vi "Benchmark SV Receive LV2012 - NI Verified - 100 Byte - 1Var.vi"() -> ()   [LabVIEW 2015]
uses:
  <vilib>/Platform/TimedLoop/XDataNode/timing_clust.ctl
  <vilib>/Platform/TimedLoop/XDataNode/nitl_modes.ctl
  <vilib>/Platform/TimedLoop/XDataNode/wakeup.ctl
  <vilib>/platform/TimedLoop/XDataNode/XDataNode.xnode
  <vilib>/Platform/TimedLoop/XDataNode/XDNodeRunTimeDep.lvlib
panel:
  out "Time":u32
  out "Counter":i32
  out "100 byte":i32[][](array[numeric])
  # "Overview:  Coding that exemplifies how to benchmark the communication of Shared Variables.\nRequirements: LabVIEW 2012 or compatible\nInstructions:\n1. Run this VI\n2. Watch the amount of time it takes to communicate on the \"Benchmark SV Send  LV2012 - NI Verified.vi\" \n3. Stop both VIs"
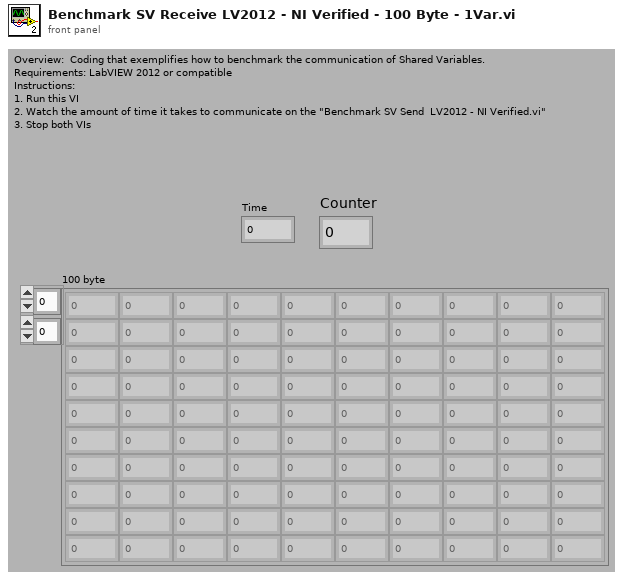
[diagram p1: front panel]
types:
  T1 = typedef "XDNodeRunTimeDep.lvlib/timing_clust.ctl" = cluster{"Expected End [f-1]":u64, "Actual End [f-1]":u64, "Finished Late? [f-1]":bool, "Expected End [i-1]":u64, "Actual End [i-1]":u64, "Finished Late? [i-1]":bool, "Expected Start [i]":u64, "Actual Start [i]":u64, "Expected Start [f]":u64, "Actual Start [f]":u64, "Source Name":string, "Structure Name":string, "Period":i64, "Deadline":i64, "Offset":i64, "Start":i64, "Priority":i32, "Timeout":i32, "Mode":T2, "Wakeup Reason":T3, "Error":errorcluster, "Source Type":string, "Secondary Source Type":string, "Global End Time":u64, "Global Start Time":u64, "Frame Duration":u64, "Iteration Duration":u64, "Assigned CPU":i32, "I/O Scan Engine Mode":u32}
  T2 = typedef "XDNodeRunTimeDep.lvlib/nitl_modes.ctl" = enum32{"No Change", "Process missed periods, maintain original phase", "Discard missed periods, maintain original phase", "Process missed periods, ignore original phase", "Discard missed periods, ignore original phase"}
  T3 = typedef "XDNodeRunTimeDep.lvlib/wakeup.ctl" = enum32{"Normal", "Aborted", "Asynchronous wakeup", "Timing source error", "Timed loop error", "Timeout"}
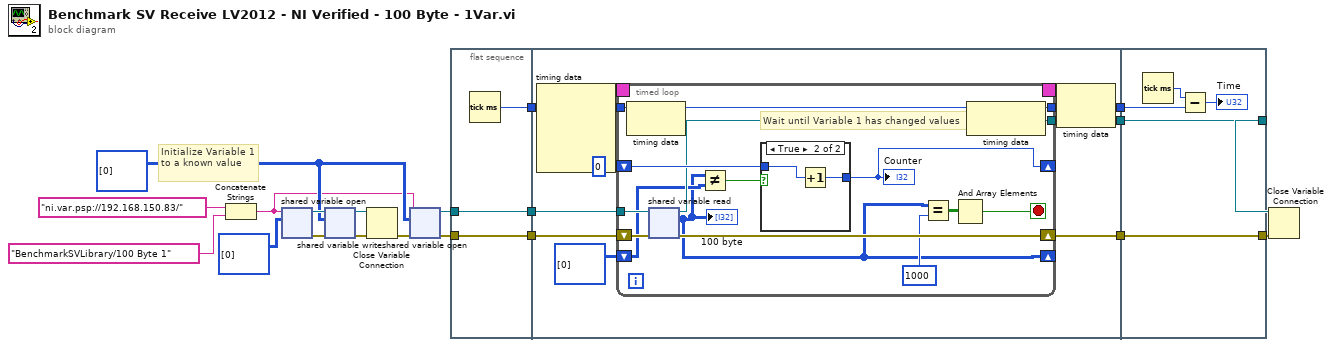
[diagram p0: block diagram]
diagram:
  w2 = i32[][] [[0]] ("1000 Byte 3")
  # "Initialize Variable 1 to a known value"
  n1 = Concatenate Strings("ni.var.psp://192.168.150.83/" ("string"), "BenchmarkSVLibrary/100 Byte 1") -> (w1:string)
  n2 = shared-variable-open(w1, i32[][] [[0]] ("appended array")) -> (w9:refnum<k21>, w7:errorcluster)  [unwired: 2 in]
  n3 = shared-variable-write(w9, w7, w2) -> (w8:refnum<k21>, w6:errorcluster)
  n4 = Close Variable Connection(8:w6, 11:w8) -> (0:w3:errorcluster)
  n5 = shared-variable-open(w1, w3, w2) -> (w13:refnum<k21>, w14:errorcluster)  [unwired: 1 in]
  n6 = flat-sequence {
    tunnel: w13 -> [w22]
    tunnel: w14 -> [w23]
    tunnel: [w23] -> w20
    tunnel: [w22] -> w19
    tunnel: [w21] -> w18
    tunnel: [w30] -> w17
    tunnel: [w29] -> w16
    tunnel: [w27] -> w15
    tunnel: w20 -> [w33]
    tunnel: w19 -> [w32]
    tunnel: w18 -> [w28]
    tunnel: w17 -> [w54]
    tunnel: w16 -> [w55]
    tunnel: w15 -> [w56]
    tunnel: [w55] -> w12
    tunnel: [w54] -> w11
    frame #0 {
      n7 = Tick Count (ms)() -> (millisecond timer value=w21:u32)
    }
    frame #1 {
      n8 = node-c288() -> (w25:T1)  [unwired: 4 in]
      n9 = timed-loop {
        shift-right: [w34] -> _
        shift-left: i32[][] [[0]] ("1000 Byte 3") -> [w38]
        shift-right: [w39] -> w30
        shift-left: w33 -> [w44]
        shift-right: [w40] -> _
        shift-left: 0 -> [w46]
        tunnel: w32 -> [w45]
        tunnel: [w43] -> w29
        tunnel: [w41] -> w27
        tunnel: w28 -> [w41]
        timing: w25 -> [_]
        timing-out: [_] -> w24
        stop <- w36 stop-if-true
        # "Wait until Variable 1 has changed values"
        n10 = node-c288() -> ()  [unwired: 1 in, 1 out]
        n11 = shared-variable-read(w45, w44) -> (w43:refnum<k21>, w39:errorcluster, w34:i32[][])  [unwired: 1 out]
        "100 byte" <- w34
        n12 = Not Equal?(x=w34, y=w38) -> (x != y?=w42:bool)
        n13 = case shown="True" w42 {
          tunnel: w46 -> [w49 w51]
          tunnel: [w49 w50] -> w40
          frame False {
          }
          frame True {
            n14 = Increment(x=w51) -> (x+1=w50:i32)
          }
        }
        "Counter" <- w40
        n15 = Equal?(x=w34, y=1000 ("Numeric")) -> (x = y?=w35:bool[][])
        n16 = And Array Elements(Boolean array=w35) -> (logical AND=w36:bool)
        n17 = node-c288() -> ()  [unwired: 1 in, 1 out]
      }
      n18 = node-c288(w24) -> ()  [unwired: 1 out]
    }
    frame #2 {
      n19 = Tick Count (ms)() -> (millisecond timer value=w58:u32)
      n20 = Subtract(x=w58, y=w56) -> (x-y=→"Time":u32)
    }
  }
  n21 = Close Variable Connection(8:w11, 11:w12) -> ()  [unwired: 1 out]
